vi "Load_from_Project.vi"(8 "error in (no error)":errorcluster, 9 "in build?":bool, 10 "sfp?":bool, 11 "Object":T1) -> (0 "error out":errorcluster, 3 "Installer out":refnum<class "Installer.lvclass">)   [LabVIEW 2020, in "Installer.lvclass"]
uses:
  <vilib>/AppBuilder/IB_Classes/Installer/Installer.lvclass
  <vilib>/AppBuilder/IB_Classes/Installer/Installer.lvclass/Installer.ctl
  <resource>/Framework/Providers/API/ItemRef.ctl
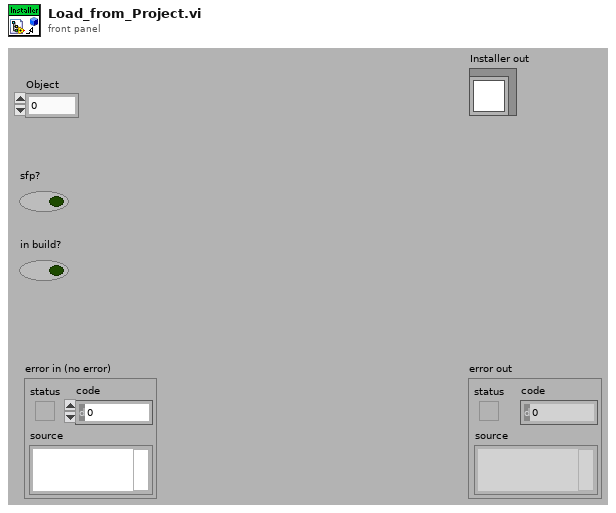
[diagram p1: front panel]
types:
  T1 = typedef "ItemRef.ctl" = u64
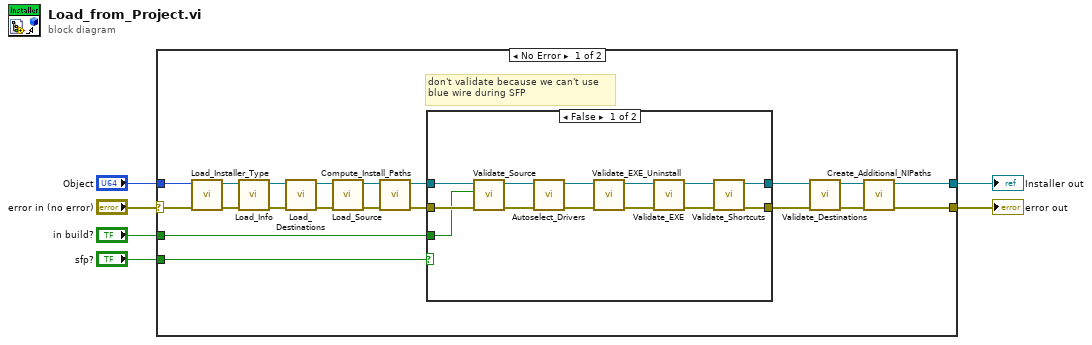
[diagram p0: block diagram]
diagram:
  n1 = case shown="No Error" "error in (no error)" {
    selector: "error in (no error)" -> [w12 w42]
    tunnel: [w15 w42] -> w4
    tunnel: [w16 _] -> w5
    tunnel: "Object" -> [w13 _]
    tunnel: "sfp?" -> [w14 _]
    tunnel: "in build?" -> [w7 _]
    frame No Error {
      # "don't validate because we can't use\nblue wire during SFP"
      n2 = call <vilib>:"Load_Installer_Type.vi"("error in (no error)"=w12, "buildObject"=w13) -> ("error out"=w25:errorcluster, "Class out"=w26:refnum<class "Installer.lvclass">)  [unwired: 1 in, 7 out]
      n3 = call-dynamic "Load_Info.vi"("error in (no error)"=w25, "Class in"=w26) -> ("error out"=w21:errorcluster, "Class out"=w22:refnum<class "Installer.lvclass">)  [unwired: 8 out]
      n4 = call <vilib>:"Load_Destinations.vi"("error in (no error)"=w21, "Installer in"=w22) -> ("error out"=w19:errorcluster, "Installer out"=w20:refnum<class "Installer.lvclass">)  [unwired: 8 out]
      n5 = call-dynamic "Load_Source.vi"("error in (no error)"=w19, "Installer in"=w20) -> ("error out"=w23:errorcluster, "Installer out"=w24:refnum<class "Installer.lvclass">)  [unwired: 8 out]
      n6 = call <vilib>:"Compute_Install_Paths.vi"("error in (no error)"=w23, "Installer in"=w24) -> ("error out"=w17:errorcluster, "Installer out"=w18:refnum<class "Installer.lvclass">)  [unwired: 8 out]
      n7 = case shown="False" w14 {
        tunnel: w18 -> [w39 w41]
        tunnel: w17 -> [w38 w40]
        tunnel: [w32 w41] -> w11
        tunnel: [w31 w40] -> w8
        tunnel: w7 -> [w37 _]
        frame False {
          n8 = call <vilib>:"Validate_Source.vi"("error in (no error)"=w38, "in build?"=w37, "Installer in"=w39) -> ("error out"=w28:errorcluster, "Installer out"=w30:refnum<class "Installer.lvclass">)  [unwired: 7 out]
          n9 = call-dynamic "Autoselect_Drivers.vi"("error in (no error)"=w28, "Installer in"=w30) -> ("error out"=w27:errorcluster, "Installer out"=w29:refnum<class "Installer.lvclass">)  [unwired: 7 in, 1 out]
          n10 = call <vilib>:"Validate_EXE_Uninstall.vi"("error in (no error)"=w27, "Installer in"=w29) -> ("error out"=w35:errorcluster, "Installer out"=w34:refnum<class "Installer.lvclass">)  [unwired: 8 in]
          n11 = call <vilib>:"Validate_EXE.vi"("error in (no error)"=w35, "Installer in"=w34) -> ("error out"=w36:errorcluster, "Installer out"=w33:refnum<class "Installer.lvclass">)  [unwired: 8 out]
          n12 = call <vilib>:"Validate_Shortcuts.vi"("error in (no error)"=w36, "Installer in"=w33) -> ("error out"=w31:errorcluster, "Installer out"=w32:refnum<class "Installer.lvclass">)  [unwired: 8 out]
        }
        frame True {
        }
      }
      n13 = call <vilib>:"Validate_Destinations.vi"("error in (no error)"=w8, "Installer in"=w11) -> ("error out"=w9:errorcluster, "Installer out"=w10:refnum<class "Installer.lvclass">)  [unwired: 8 in]
      n14 = call <vilib>:"Create_Additional_NIPaths.vi"("error in (no error)"=w9, "Installer in"=w10) -> ("error out"=w15:errorcluster, "Installer out"=w16:refnum<class "Installer.lvclass">)  [unwired: 8 out]
    }
    frame Error {
    }
  }
  "error out" <- w4
  "Installer out" <- w5
